vi "GetCursorPos.vi"(8 "错误输入（无错误）":errorcluster) -> (0 "错误输出":errorcluster, 2 "Pos":cluster{"X":i32, "Y":i32}, 3 "布尔":bool)   [LabVIEW 2018, in "Win32API.lvlib"]
uses:
  Win32API.lvlib
  user32.dll
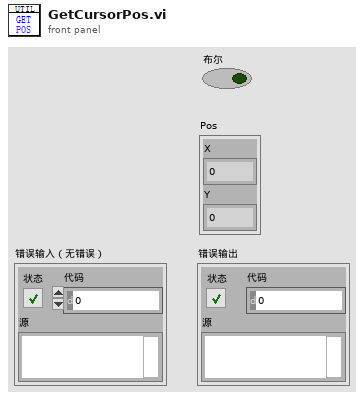
[diagram p1: front panel]
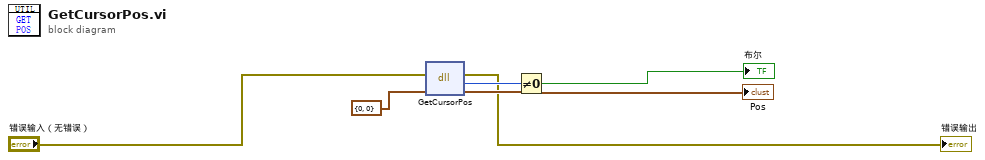
[diagram p0: block diagram]
diagram:
  n1 = dll-call lib="user32.dll" fn="GetCursorPos"(error in="错误输入（无错误）", "Pos"=cluster{"X":i32, "Y":i32} {"X"=0, "Y"=0}) -> (error out=→"错误输出":errorcluster, "Result"=w3:i32, "Pos"=→"Pos":cluster{"X":i32, "Y":i32})  [unwired: 2 in, 1 out]
  n2 = Not Equal To 0?(x=w3) -> (x != 0?=→"布尔":bool)
